vi "GT Ln XYZACUVWWN.vi"(0 "cardNum":i16, 1 "synVel":dbl, 2 "velEnd":dbl, 3 "fifo":i16, 5 "crd":i16, 7 "pPos":i32, 9 "posMask":i16, 11 "error in (no error)":errorcluster caption="错误输入（无错误）", 12 "synAcc":dbl, 13 "segNum":i32) -> (4 "function return":i16, 8 "pPos out":i32, 15 "error out":errorcluster caption="错误输出")   [LabVIEW 2020, in "gts.lvlib"]
doc: "GT_API GT_LnXYZACUVWWN(short cardNum,short crd,long *pPos,short posMask,double synVel,double synAcc,double velEnd=0,long segNum=0,short fifo=0);"
uses:
  gts.lvlib
  dll/32bit/multi_card/gts.dll
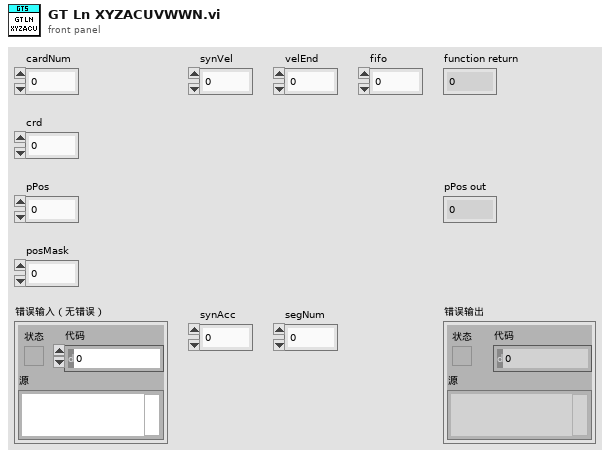
[diagram p1: front panel]
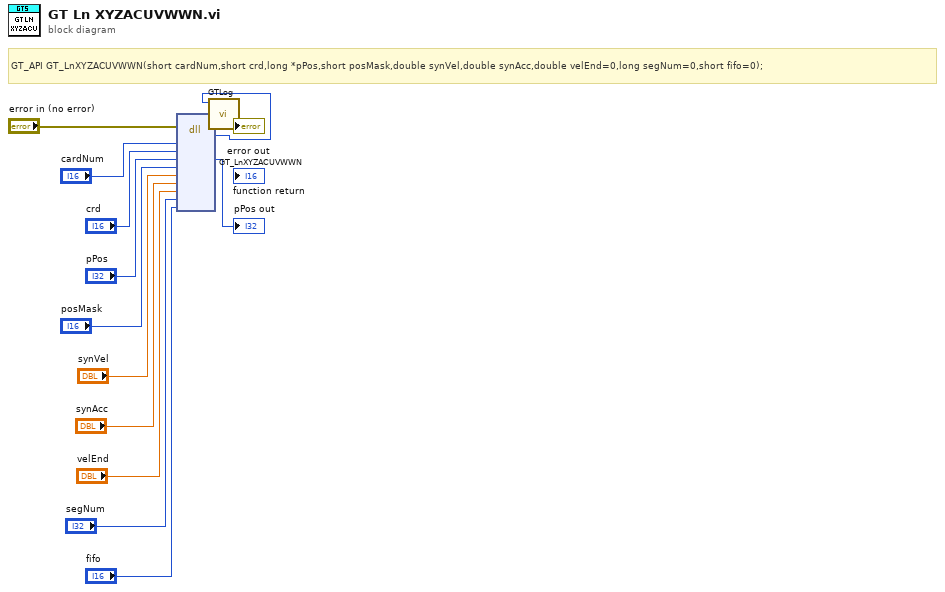
[diagram p0: block diagram]
diagram:
  # "GT_API GT_LnXYZACUVWWN(short cardNum,short crd,long *pPos,short posMask,double synVel,double synAcc,double velEnd=0,long segNum=0,short fifo=0);"
  n1 = dll-call lib="C:/1228/dll/32bit/multi_card/gts.dll" fn="GT_LnXYZACUVWWN"(error in="error in (no error)", "cardNum"="cardNum", "crd"="crd", "pPos"="pPos", "posMask"="posMask", "synVel"="synVel", "synAcc"="synAcc", "velEnd"="velEnd", "segNum"="segNum", "fifo"="fifo") -> (error out=w3:errorcluster, w1:i16, "pPos"=→"pPos out":i32)  [unwired: 10 in, 1 out]
  n2 = call "GTLog.vi"("error in (no error)"=w3, "Numeric"=w1) -> ("error out"=→"error out":errorcluster)  [unwired: 9 in]
